vi "sta_error calculator (SubVI).vi"(8 "에러 입력(에러 없음)":errorcluster, 9 "targets":dbl[](array[numeric]), 10 "predictions":dbl[](array[numeric]), 11 "error type":u16(ring) items=["RMSE", "MAE", "RTE", "4", "3", "2", "1"]) -> (0 "에러 출력":errorcluster, 1 "ans array":dbl[](array[numeric]), 2 "ans":dbl, 3 "참조 번호 출력":refnum<k35>)   [LabVIEW 2018]
uses:
  PythonConfigGlobal.vi
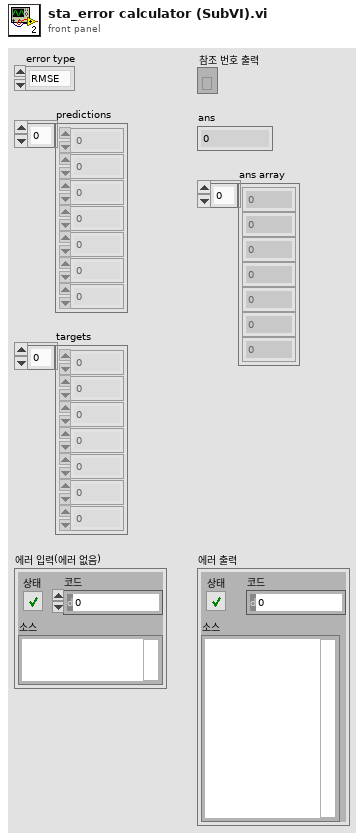
[diagram p1: front panel]
types:
  T1 = cluster{"session out":refnum<k35>, "appended path":path}
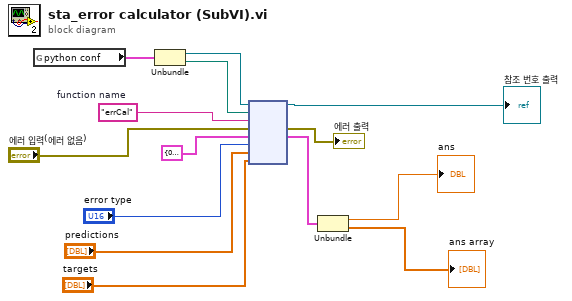
[diagram p0: block diagram]
diagram:
  w8 = "errCal"  # function name
  n1 = global read "PythonConfigGlobal.vi" "python conf"() -> (w3:T1)
  n2 = Unbundle(w3) -> ("session out"=w7:refnum<k35>, "appended path"=w6:path)
  n3 = node(w7, w6, w8, "에러 입력(에러 없음)", cluster{"ans":dbl, "ans array":dbl[]} {"ans"=0.0, "ans array"=[0.36725715488541333, 0.14005920629024704, 0.9817361238610962, 0.8216506096978233, 0.2843249179113163, 0.9126494110409356, 0.5532123513806231, 0.32885422219737315, 0.3695092956766908, 0.6935862547181748, 0.9804690731159791, 0.46595340165445087, 0.3431042302406597, 0.23251300146575948, 0.13629290128896843, 0.28811629007988165, 0.22561879575785726, 0.5634047300816905, 0.2696760726361178, 0.357634152983505, 0.128474351012541, 0.6743975440725758, 0.009204231819711417, 0.11444653507567093, 0.9937134470100775, 0.823316238165889, 0.08347131904930505, 0.8573305517223413, 0.663002360735844, 0.30365215533797807]}, "error type", "predictions", "targets") -> (→"참조 번호 출력":refnum<k35>, →"에러 출력":errorcluster, w9:cluster{"ans":dbl, "ans array":dbl[]})  [unwired: 3 in, 2 out]
  n4 = Unbundle(w9) -> ("ans"=→"ans":dbl, "ans array"=→"ans array":dbl[])
